vi "main.vi"() -> ()   [LabVIEW 2018]
doc: "Replays a chess game using PGN game file from chess.com."
uses:
  code/board/board_actions.ctl
panel:
  out "move":string
  in  "pause":bool
  in  "prev":bool
  in  "next":bool
  in  "play":bool
  in  "reset":bool
  in  "stop":bool
  out "board":picture[][](array[picture])
  in  "board actions (reset)":T1=enum."reset"
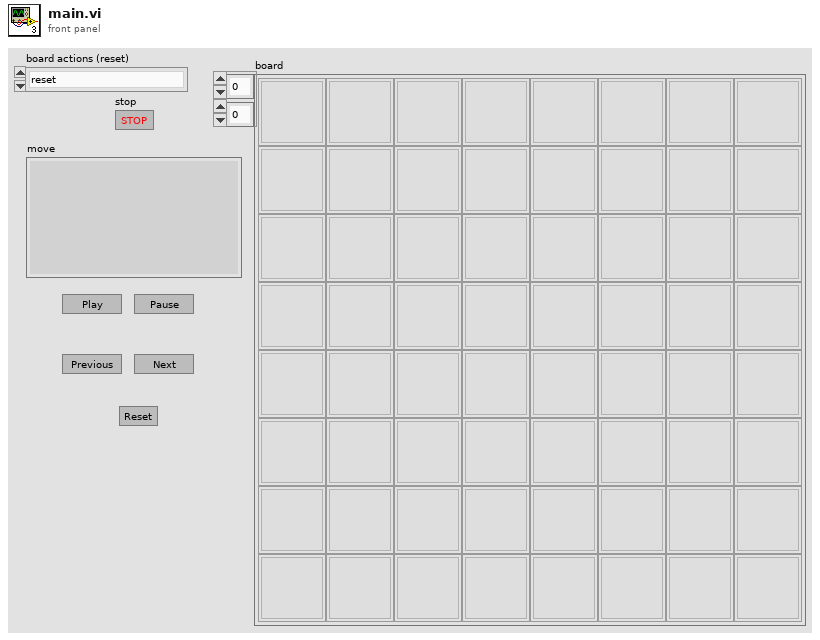
[diagram p1: front panel]
types:
  T1 = typedef "board_actions.ctl" = enum16{"move", "reset"}
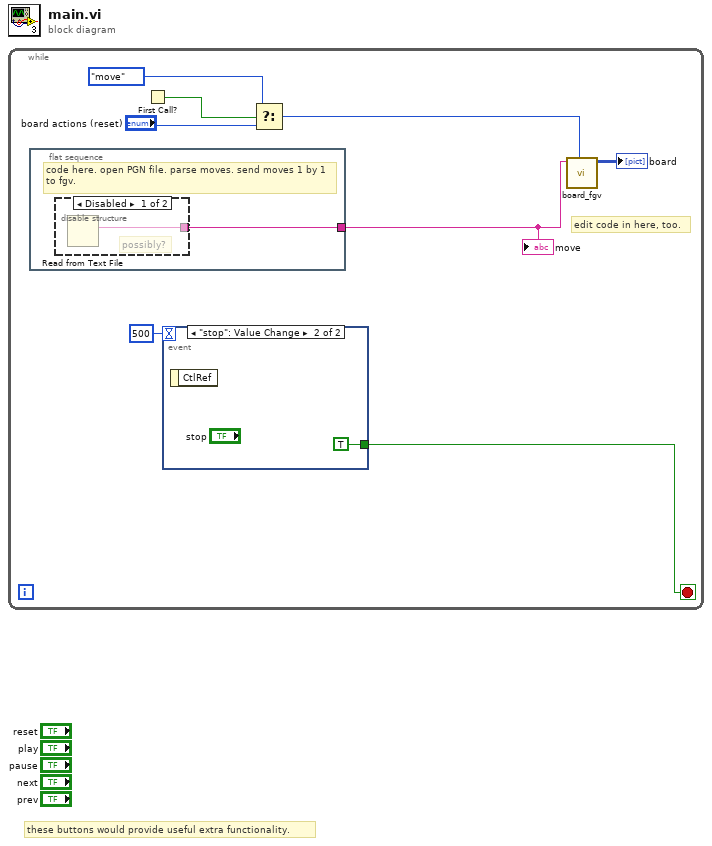
[diagram p0: block diagram]
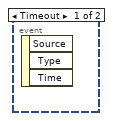
[diagram p2: hidden frame]
diagram:
  # "these buttons would provide useful extra functionality."
  n1 = while {
    stop <- w2 stop-if-true
    # "edit code in here, too."
    n2 = flat-sequence {
      tunnel: [w10] -> w3
      frame #0 {
        # "code here. open PGN file. parse moves. send moves 1 by 1 to fgv."
        n3 = disable-structure shown="Disabled" {
          disable-tunnel: [w11 _] -> w10
          frame Disabled {
            # "possibly?"
            n4 = Read from Text File() -> (text=w11:string)  [unwired: 4 in, 3 out]
          }
          frame Enabled {
          }
        }
      }
    }
    n5 = First Call?() -> (First Call?: T/F=w8:bool)
    n6 = event shown="[1] \"stop\": Value Change" {
      selector: _ -> [_ _]
      dyn-events: _ -> [_ _]
      timeout: 500 -> [_ _]
      tunnel: [_ TRUE] -> w2
      event Timeout {
        n7 = event-data() -> ()  [unwired: 1 in, 3 out]
      }
      event "stop": Value Change {
        n8 = event-data() -> ()  [unwired: 1 in, 1 out]
      }
    }
    n9 = Select(t=board_actions."move" ("board actions (reset)"), s=w8, f="board actions (reset)") -> (s? t:f=w5:T1)
    n10 = call "board_fgv.vi"("board actions (reset)"=w5, "move"=w3) -> ("board"=→"board":picture[][])  [unwired: 9 in]
    "move" <- w3
  }
